vi "Text File_Change the Header.vi"(8 "error in (no error)":errorcluster caption="에러 입력(에러 없음)", 11 "참조 출력":refnum<class "Text File.lvclass">) -> (0 "error out":errorcluster caption="에러 출력", 3 "참조 출력 2":refnum<class "Text File.lvclass">)   [LabVIEW 2020, in "Text File.lvclass"]
uses:
  Text File.lvclass
  SubVIs/Waveform Editor/Controls/(Ctrl)Waveform Editor_WF List.ctl
  Waveform Obj/Waveform Obj.lvclass
  Haptic IC Class/Haptic IC/Controls/(Ctrl)IC Type.ctl
  Text File.lvclass/Text File.ctl
  Haptic IC Class/DW7800/DW7800.lvclass
  Haptic IC Class/DW7802/DW7802.lvclass
  Haptic IC Class/DW7912/DW7912.lvclass
  Haptic IC Class/DW7914/DW7914.lvclass
  Haptic IC Class/Haptic IC/Haptic IC.lvclass/Haptic IC.ctl
  Waveform Obj/Waveform Obj.lvclass/Waveform Obj.ctl
  Accessors/Read Text_Data.vi
  Accessors/Read Text_Format.vi
  Accessors/Read Text_ic type.vi
  Haptic IC Class/Haptic IC/Accessors/Write ic type.vi
  Accessors/Read Text_Sampling Rate.vi
  Waveform Obj/Accessors/Read sampling rate.vi
  Waveform Obj/Accessors/Write sampling rate.vi
  Accessors/Write Text_Header.vi
  Accessors/Write Text_Data.vi
  Haptic IC Class/Haptic IC/Haptic IC.lvclass
panel:
  out "숫자형 2":i32
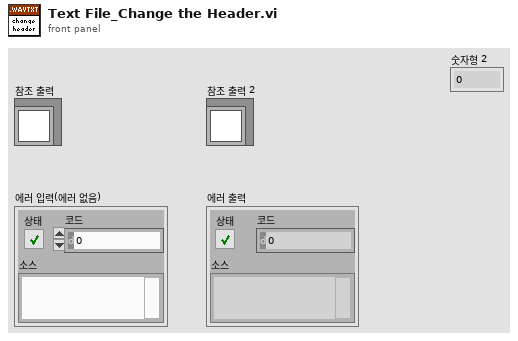
[diagram p1: front panel]
types:
  T1 = typedef "(Ctrl)Waveform Editor_WF List.ctl" = cluster{"Name":string, "WF Seq":refnum<class "Waveform Obj.lvclass">[]}
  T2 = typedef "Haptic IC.lvclass/(Ctrl)IC Type.ctl" = enum8{"DW7800", "DW7802", "DW7912", "DW7914"}
  T3 = cluster{"TXT_Radix":enum16{"BIN", "DEC", "HEX"}, "TXT_Prefix":bool, "TXT_Delimiter":string, "TXT_End of LIne":enum16{"EOL (\\r\\n)", "LF (\\n)"}, "TXT_EOL+Delimiter":bool, "TXT_Number per Line":i32}
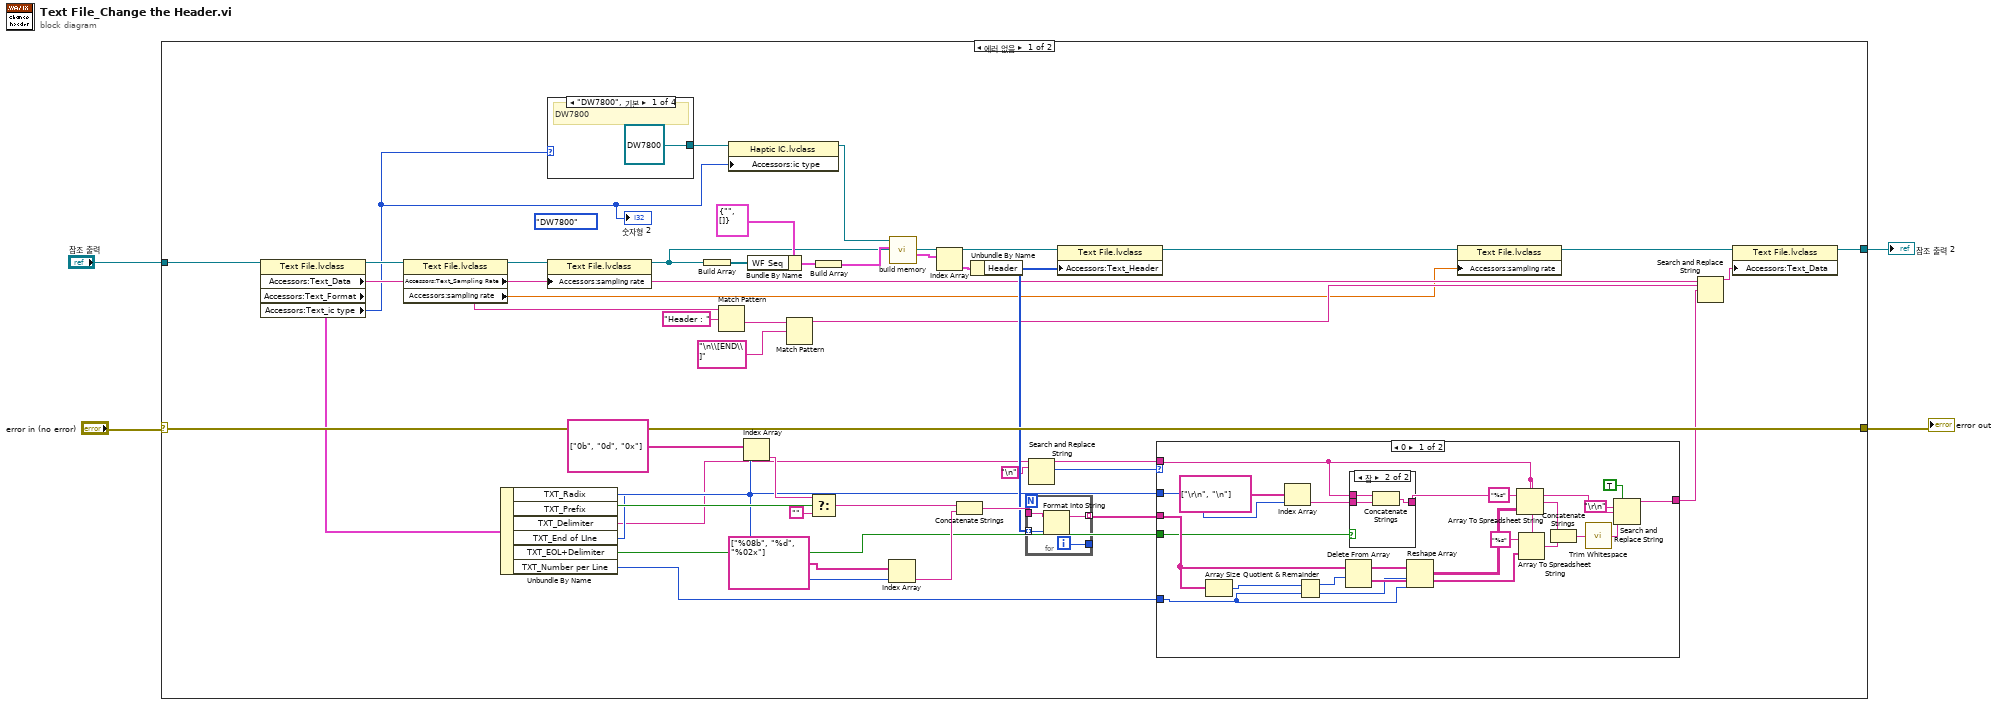
[diagram p0: block diagram]
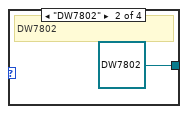
[diagram p2: hidden frame]
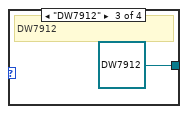
[diagram p3: hidden frame]
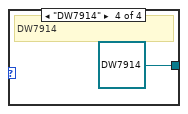
[diagram p4: hidden frame]
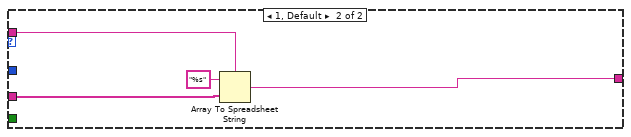
[diagram p6: hidden frame]
diagram:
  n1 = case shown="에러 없음" "error in (no error)" {
    selector: "error in (no error)" -> [w48 w89]
    tunnel: [w48 w89] -> w3
    tunnel: "참조 출력" -> [w47 w88]
    tunnel: [w8 w88] -> w1
    frame No Error {
      (unwired) (Ctrl)IC_Type."DW7800" ("Text_ic type")
      n2 = property class="Text File.lvclass"(reference=w47) -> (reference out=w40:refnum<class "Text File.lvclass">, "Accessors:Text_Data"=w20:string, "Accessors:Text_Format"=w39:T3, "Accessors:Text_ic type"=w5:T2)  [unwired: 1 in, 1 out]
      "숫자형 2" <- w5
      n3 = property class="Text File.lvclass"(reference=w40) -> (reference out=w13:refnum<class "Text File.lvclass">, "Accessors:Text_Sampling Rate"=w12:i32, "Accessors:sampling rate"=w11:dbl)  [unwired: 1 in, 1 out]
      n4 = Unbundle By Name(w39) -> ("TXT_Radix"=w33:enum16{"BIN", "DEC", "HEX"}, "TXT_Prefix"=w35:bool, "TXT_Delimiter"=w15:string, "TXT_End of LIne"=w25:enum16{"EOL (\\r\\n)", "LF (\\n)"}, "TXT_EOL+Delimiter"=w24:bool, "TXT_Number per Line"=w16:i32)
      n5 = property class="Text File.lvclass"(reference=w13, "Accessors:sampling rate"=w12) -> (reference out=w14:refnum<class "Text File.lvclass">)  [unwired: 1 in, 1 out]
      n6 = case shown="\"DW7800\", 기본" w5 {
        tunnel: [refnum<class "DW7800.lvclass"> refnum ("DW7800.lvclass") refnum<class "DW7802.lvclass"> refnum ("DW7802.lvclass") refnum<class "DW7912.lvclass"> refnum ("DW7912.lvclass") refnum<class "DW7914.lvclass"> refnum ("DW7914.lvclass")] -> w10
        frame "DW7800", Default {
          # "DW7800"
        }
        frame "DW7802" {
          # "DW7802"
        }
        frame "DW7912" {
          # "DW7912"
        }
        frame "DW7914" {
          # "DW7914"
        }
      }
      n7 = Build Array(w14) -> (w45:refnum<class "Text File.lvclass">[])
      n8 = Match Pattern(string=w20, regular expression="Header : " ("정규식")) -> (after substring=w22:string)  [unwired: 1 in, 3 out]
      n9 = property class="Haptic IC.lvclass"(reference=w10, "Accessors:ic type"=w5) -> (reference out=w6:refnum<class "Haptic IC.lvclass">)  [unwired: 1 in, 1 out]
      n10 = Index Array(array=string[] ["0b", "0d", "0x"], index=w33) -> (element=w36:string)
      n11 = Bundle By Name(cluster=T1 {"Name"="", "WF Seq"=[]} ("WF List"), "WF Seq"=w45) -> (w44:T1)
      n12 = Match Pattern(string=w22, regular expression="\n\\[END\\]" ("정규식")) -> (before substring=w19:string)  [unwired: 1 in, 3 out]
      n13 = Select(t=w36, s=w35, f="") -> (s? t:f=w32:string)
      n14 = Build Array(w44) -> (w43:T1[])
      n15 = Index Array(array=string[] ["%08b", "%d", "%02x"], index=w33) -> (element=w31:string)
      n16 = call-dynamic "build memory.vi"("WF List"=w43, "Haptic IC 입력"=w6) -> ("memory data by wf"=w42:cluster{"Header":u8[], "Data":u8[]}[])  [unwired: 6 in, 3 out]
      n17 = Index Array(array=w42) -> (element=w41:cluster{"Header":u8[], "Data":u8[]})  [unwired: 1 in]
      n18 = Concatenate Strings(w32, w31) -> (w30:string)
      n19 = Unbundle By Name(w41) -> ("Header"=w29:u8[])
      n20 = for {
        tunnel: w30 -> [w87]
        tunnel: [w86] -> w27 mode=indexing
        tunnel: [w85] -> _
        tunnel: w29 -> [w84] mode=indexing
        i -> [w85]
        n21 = Format Into String(format string=w87, w84) -> (resulting string=w86:string)  [unwired: 2 in, 1 out]
      }
      n22 = Search and Replace String(input string=w15, search string="\n") -> (number of replacements=w26:i32)  [unwired: 6 in, 3 out]
      n23 = property class="Text File.lvclass"(reference=w14, "Accessors:Text_Header"=w29) -> (reference out=w17:refnum<class "Text File.lvclass">)  [unwired: 1 in, 1 out]
      n24 = case shown="0" w26 {
        tunnel: w27 -> [w60 w82]
        tunnel: [w57 w81] -> w18
        tunnel: w15 -> [w61 w80]
        tunnel: w25 -> [w59 _]
        tunnel: w24 -> [w58 _]
        tunnel: w16 -> [w54 _]
        frame 0 {
          n25 = Array Size(array=w60) -> (size(s)=w55:i32)
          n26 = Index Array(array=string[] ["\r\n", "\n"], index=w59) -> (element=w62:string)
          n27 = Quotient & Remainder(x=w55, y=w54) -> (x-y*floor(x/y)=w53:i32, floor(x/y)=w56:i32)
          n28 = Delete From Array(array=w60, length=w53) -> (deleted portion=w67:string[], array with subset deleted=w73:string[])  [unwired: 1 in]
          n29 = case shown="참" w58 {
            tunnel: w62 -> [w76 w79]
            tunnel: w61 -> [_ w78]
            tunnel: [w76 w77] -> w69
            frame False {
            }
            frame True {
              n30 = Concatenate Strings(w78, w79) -> (w77:string)
            }
          }
          n31 = Reshape Array(w73, w56, w54) -> (w72:string[][])
          n32 = Array To Spreadsheet String(delimiter (Tab)=w61, array=w72, 3:"%s" ("포맷 문자열")) -> (spreadsheet string=w66:string)
          n33 = Array To Spreadsheet String(delimiter (Tab)=w61, array=w67, 3:"%s" ("포맷 문자열")) -> (spreadsheet string=w65:string)
          n34 = Concatenate Strings(w66, w65) -> (w64:string)
          n35 = call <vilib>:"Trim Whitespace.vi"("string"=w64) -> ("trimmed string"=w63:string)  [unwired: 1 in]
          n36 = Search and Replace String(replace all?=TRUE ("모두 대체? (거짓)"), input string=w63, search string="\r\n" ("검색 문자열"), replace string=w69) -> (result string=w57:string)  [unwired: 4 in, 3 out]
        }
        frame 1, Default {
          n37 = Array To Spreadsheet String(delimiter (Tab)=w80, array=w82, 3:"%s" ("포맷 문자열")) -> (spreadsheet string=w81:string)
        }
      }
      n38 = property class="Text File.lvclass"(reference=w17, "Accessors:sampling rate"=w11) -> (reference out=w9:refnum<class "Text File.lvclass">)  [unwired: 1 in, 1 out]
      n39 = Search and Replace String(input string=w20, search string=w19, replace string=w18) -> (result string=w7:string)  [unwired: 5 in, 3 out]
      n40 = property class="Text File.lvclass"(reference=w9, "Accessors:Text_Data"=w7) -> (reference out=w8:refnum<class "Text File.lvclass">)  [unwired: 1 in, 1 out]
    }
    frame Error {
    }
  }
  "참조 출력 2" <- w1
  "error out" <- w3
